vi "Get Apriltag Number from Image.vi"(9 "Corners":cluster{"X":sgl, "Y":sgl}[](array[cluster]), 11 "Image":T1(plugin-control)) -> (3 "AprilTag#":i32)   [LabVIEW 2023]
uses:
  <vilib>/vision/NI_Vision_Development_Module.lvlib
panel:
  in  "Range":cluster{"Lower value":sgl, "Upper value":sgl}={"Lower value"=128.0, "Upper value"=255.0}
  out "Apriltag":T1(plugin-control)
  in  "Tag 21":u32
  in  "Tag 20":u32
  in  "Tag 19":u32
  in  "Tag 18":u32
  in  "Tag 17":u32
  in  "Tag 16":u32
  in  "Tag 15":u32
  in  "Tag 14":u32
  in  "Tag 13":u32
  in  "Tag 12":u32
  in  "Tag 11":u32
  in  "Tag 10":u32
  in  "Tag 9":u32
  in  "Tag 8":u32
  in  "Tag 7":u32
  in  "Tag 6":u32
  in  "Tag 4":u32
  in  "Tag 2":u32
  in  "Tag1":u32
  in  "Tag 5":u32
  in  "Tag 3":u32
  in  "Tag 22":u32
  out "Bool Array":bool[][](array[boolean])
  out "Array 2":u8[][](array[numeric])
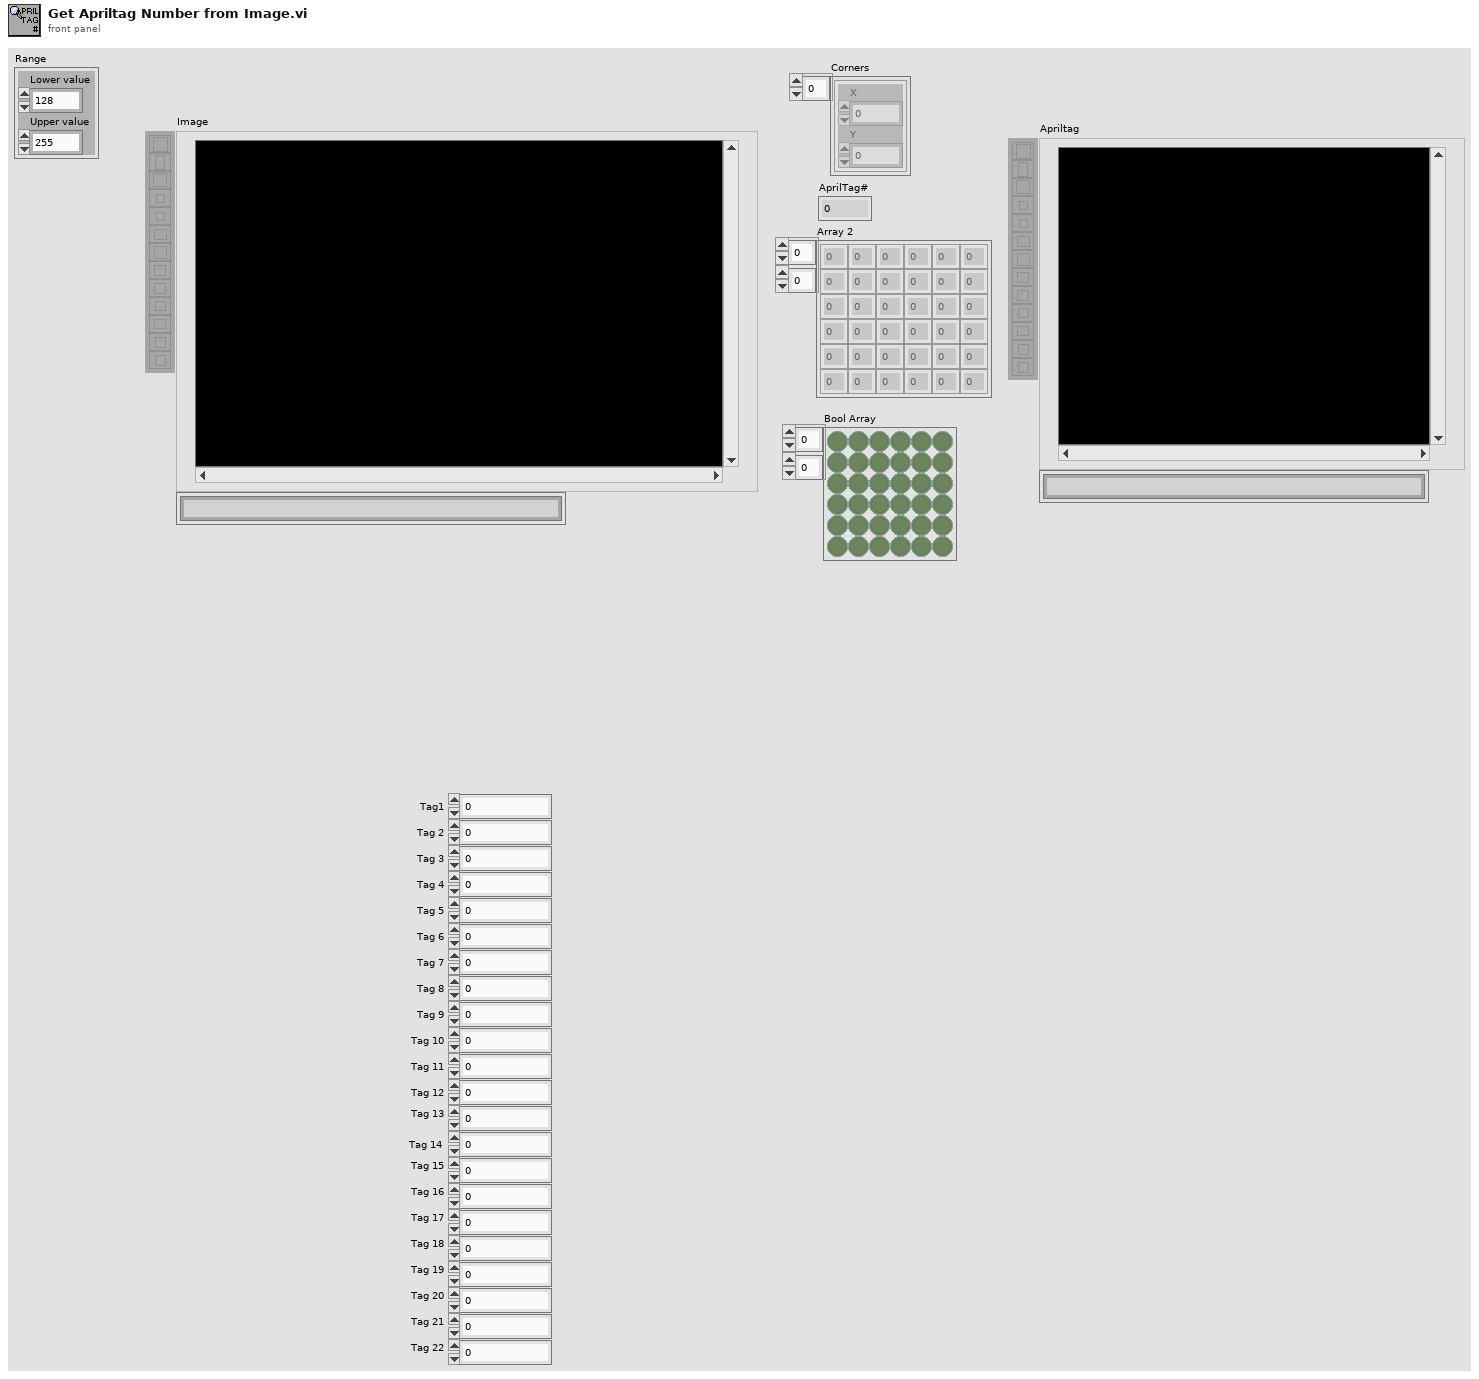
[diagram p1: front panel]
types:
  T1 = typedef "IMAQ Image.ctl" = refnum<image>
  T2 = typedef "Image Type" = u32
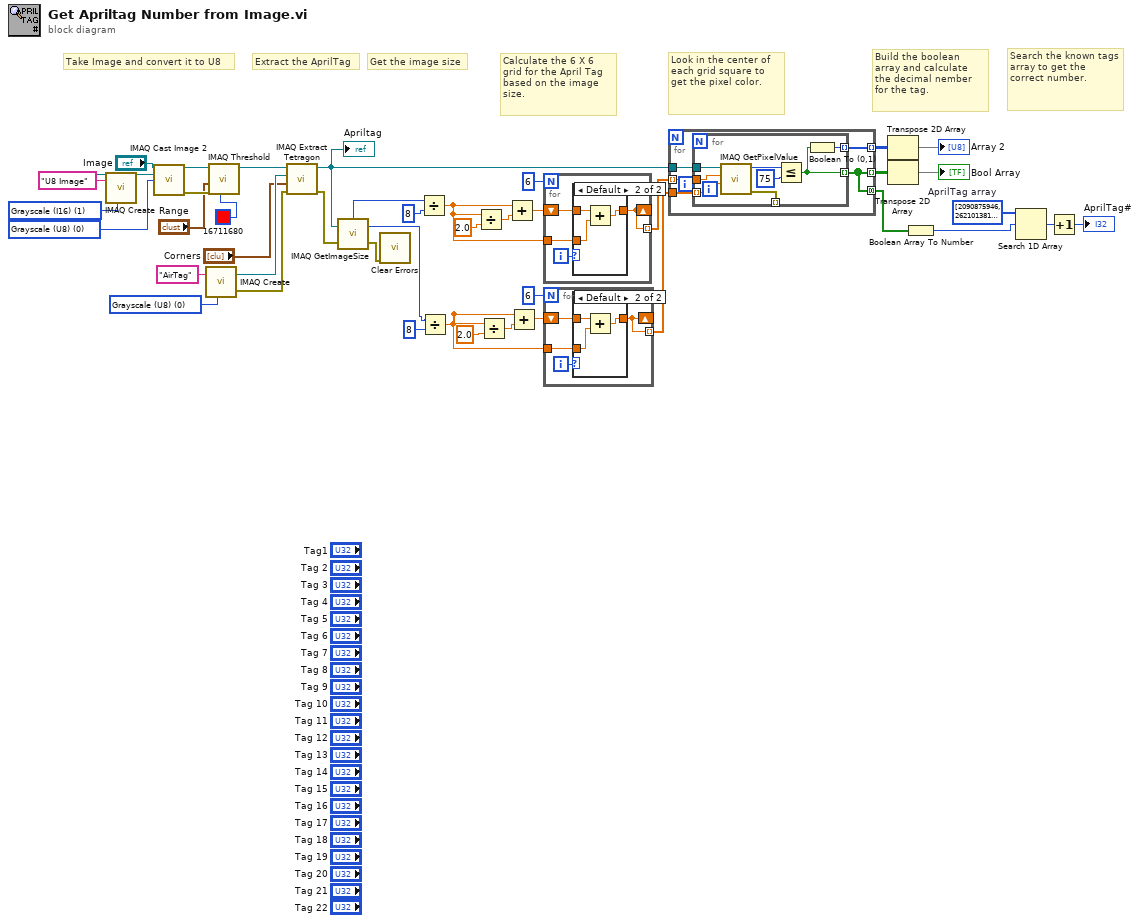
[diagram p0: block diagram]
diagram:
  w11 = T2 0 items=["Grayscale (U8)", "Grayscale (I16)", "Grayscale (SGL)", "Complex (CSG)", "RGB (U32)", "HSL (U32)", "RGB (U64)", "Grayscale (U16)"] ("Image Type")
  w17 = u32[] [2090875946, 2621013818, 702899106, 3538358024, 1663594000, 2908175739, 3842209527, 1632389581, 469213657, 154307819, 610517857, 3321664829, 2540025641, 780983953, 3474046093, 2055835671, 1884137891, 4040607285, 216557965, 1333074778, 3211662662, 103108830]  # AprilTag array
  w29 = T2 0 items=["Grayscale (U8)", "Grayscale (I16)", "Grayscale (SGL)", "Complex (CSG)", "RGB (U32)", "HSL (U32)", "RGB (U64)", "Grayscale (U16)"] ("Image Type")
  w32 = T2 1 items=["Grayscale (U8)", "Grayscale (I16)", "Grayscale (SGL)", "Complex (CSG)", "RGB (U32)", "HSL (U32)", "RGB (U64)", "Grayscale (U16)"] ("Image Type")
  # "Search the known tags array to get the correct number."
  # "Build the boolean array and calculate the decimal nember for the tag."
  # "Look in the center of each grid square to get the pixel color."
  # "Calculate the 6 X 6 grid for the April Tag based on the image size."
  # "Get the image size"
  # "Extract the AprilTag"
  # "Take Image and convert it to U8"
  n1 = call "IMAQ Create"("Image Name"="U8 Image", "Image Type"=w32) -> ("New Image"=w31:T1)  [unwired: 2 in, 2 out]
  n2 = call "IMAQ Cast Image 2"("Image Src"="Image", "Image Dst"=w31, "Image Type"=w29) -> ("Image Dst Out"=w5:T1, "error out"=w3:errorcluster)  [unwired: 11 in]
  n3 = call "IMAQ Create"("Image Name"="AirTag" ("string"), "Image Type"=w11) -> ("New Image"=w10:T1, "error out"=w9:errorcluster)  [unwired: 2 in, 1 out]
  n4 = call "IMAQ Threshold"("Replace Value"=u32 16711680, "error in (no error)"=w3, "Range"="Range", "Image Src"=w5) -> ("Image Dst Out"=w4:T1)  [unwired: 6 in, 1 out]
  n5 = call-poly "IMAQ Extract Tetragon"("error in (no error)"=w9, "Tetragon"="Corners", "Image Dst"=w10, "Image Src"=w4) -> ("error out"=w6:errorcluster, "Image Dst Out"=w7:T1)  [unwired: 6 in]
  "Apriltag" <- w7
  n6 = call "IMAQ GetImageSize"("Image"=w7, "error in (no error)"=w6) -> ("Y Resolution"=w15:i32, "X Resolution"=w16:i32, "error out"=w28:errorcluster)  [unwired: 2 in]
  n7 = call <vilib>:"Clear Errors.vi"("error in (no error)"=w28) -> ()  [unwired: 5 in, 2 out]
  n8 = Divide(x=w16, y=8) -> (x/y=w14:dbl)
  n9 = Divide(x=w15, y=8) -> (x/y=w13:dbl)
  n10 = Divide(x=w14, y=2.0) -> (x/y=w41:dbl)
  n11 = Divide(x=w13, y=2.0) -> (x/y=w38:dbl)
  n12 = Add(x=w14, y=w41) -> (x+y=w37:dbl)
  n13 = Add(x=w13, y=w38) -> (x+y=w34:dbl)
  n14 = for {
    N: 6 -> [_]
    tunnel: w14 -> [w45]
    tunnel: [w44] -> w27 mode=indexing
    shift-right: [w44] -> _
    shift-left: w37 -> [w46]
    i -> [w47]
    n15 = case shown="Default" w47 {
      tunnel: w46 -> [w48 w51]
      tunnel: [w48 w50] -> w44
      tunnel: w45 -> [_ w49]
      frame 0 {
      }
      frame Default {
        n16 = Add(x=w51, y=w49) -> (x+y=w50:dbl)
      }
    }
  }
  n17 = for {
    N: 6 -> [_]
    tunnel: w13 -> [w53]
    shift-right: [w52] -> _
    shift-left: w34 -> [w54]
    tunnel: [w52] -> w26 mode=indexing
    i -> [w55]
    n18 = case shown="Default" w55 {
      tunnel: w54 -> [w56 w59]
      tunnel: [w56 w58] -> w52
      tunnel: w53 -> [_ w57]
      frame 0 {
      }
      frame Default {
        n19 = Add(x=w59, y=w57) -> (x+y=w58:dbl)
      }
    }
  }
  n20 = for {
    tunnel: w7 -> [w64]
    tunnel: w27 -> [w63] mode=indexing
    tunnel: [w60] -> w23 mode=indexing
    tunnel: w26 -> [w62]
    tunnel: [w61] -> w25 mode=indexing
    tunnel: [w60] -> w21 mode=concatenating
    n21 = for {
      tunnel: w64 -> [w72]
      tunnel: [w68] -> w60 mode=indexing
      tunnel: w63 -> [w71]
      tunnel: w62 -> [w70] mode=indexing
      tunnel: [w66] -> w61 mode=indexing
      tunnel: [w65] -> _ mode=indexing
      n22 = call "IMAQ GetPixelValue"("Image"=w72, "X Coordinate"=w71, "Y Coordinate"=w70) -> ("Pixel Value (U8)"=w67:u8, "error out"=w65:errorcluster)  [unwired: 3 in, 3 out]
      n23 = Less Or Equal?(x=w67, y=u8 75) -> (x <= y?=w68:bool)
      n24 = Boolean To (0,1)(Boolean=w68) -> (0, 1=w66:i16)
    }
  }
  n25 = Transpose 2D Array(2D array=w25) -> (transposed array=→"Array 2":i16[][])
  n26 = Transpose 2D Array(2D array=w23) -> (transposed array=→"Bool Array":bool[][])
  n27 = Boolean Array To Number(Boolean array=w21) -> (number=w20:u32)
  n28 = Search 1D Array(1D array=w17, element=w20) -> (index of element=w19:i32)  [unwired: 1 in]
  n29 = Increment(x=w19) -> (x+1=→"AprilTag#":i32)
